vi "testRSASign&Verify.vi"(8 "error in (no error)":errorcluster, 11 "TestCase in":refnum<class "TestRSA.lvclass">) -> (0 "error out":errorcluster, 3 "TestCase out":refnum<class "TestRSA.lvclass">)   [LabVIEW 2021, in "TestRSA.lvclass"]
uses:
  TestRSA.lvclass
  TestRSA.lvclass/TestRSA.ctl
  <vilib>/addons/_JKI Toolkits/VI Tester/TestCase.llb/TestCase.lvclass
  Asymmetric Encryption/dotNET Crypto Asymmetric Encryption.lvlib
  Key Management/dotNET Crypto Key Management.lvlib
  Asymmetric Encryption/RSA/HashingAlgorithm.ctl
  Utility/dotNET Crypto Utility.lvlib
  Asymmetric Encryption/RSA/RSASignaturePadding.ctl
  C:/Program Files (x86)/National Instruments/LabVIEW 2021/vi.lib/addons/_JKI Toolkits/VI Tester/TestCase.llb/TestCase.lvclass
  C:/LabVIEW Working Directory/labview-keystore/Unit Tests/TestRSA/TestRSA.lvclass
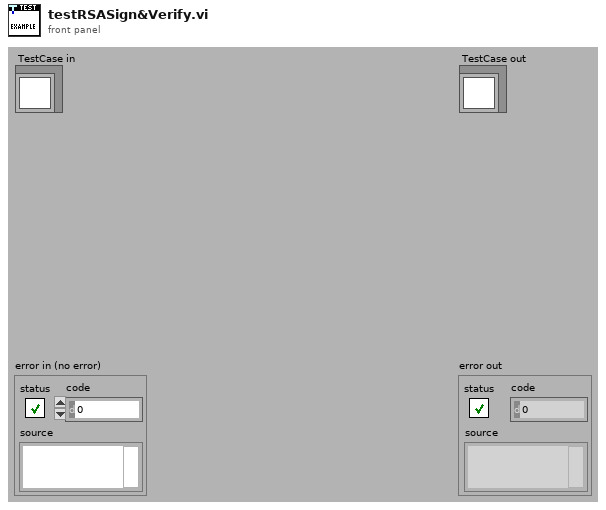
[diagram p1: front panel]
types:
  T1 = typedef "dotNET Crypto Asymmetric Encryption.lvlib/RSASignaturePadding.ctl" = enum16{"Pkcs1", "Pss"}
  T2 = typedef "dotNET Crypto Utility.lvlib/HashingAlgorithm.ctl" = enum16{"MD5", "SHA1", "SHA256", "SHA384", "SHA512"}
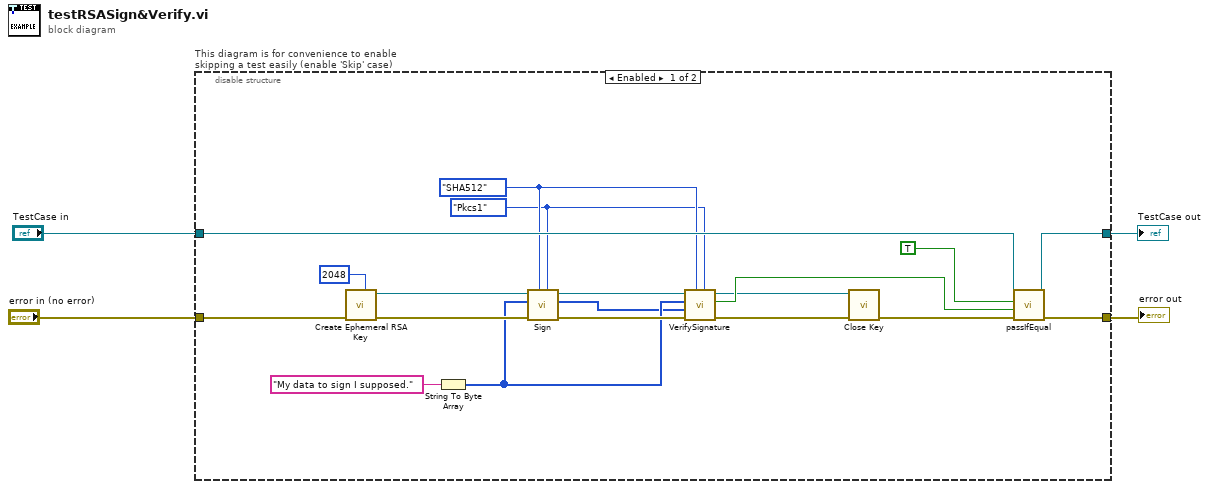
[diagram p0: block diagram]
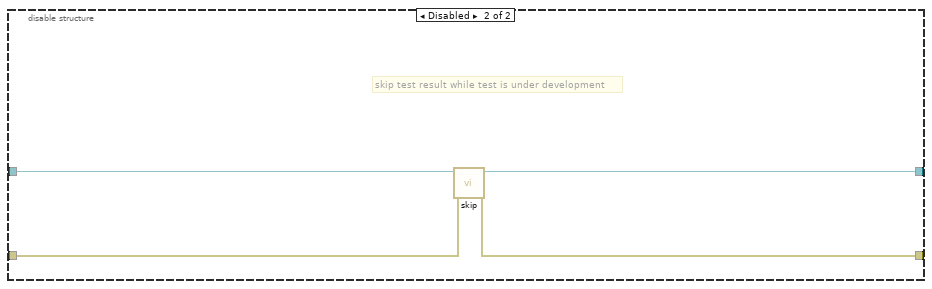
[diagram p2: hidden frame]
diagram:
  n1 = disable-structure "This diagram is for convenience to enable skipping a test easily (enable 'Skip' case)" shown="Enabled" {
    disable-tunnel: "TestCase in" -> [w23 w27]
    disable-tunnel: [w22 w25] -> w1
    disable-tunnel: [w21 w26] -> w3
    disable-tunnel: "error in (no error)" -> [w20 w24]
    frame Enabled {
      w16 = RSASignaturePadding."Pkcs1" ("RSASignPadding")
      w17 = HashingAlgorithm."SHA512" ("HashingAlgorithm")
      n2 = call "Create Ephemeral RSA Key.vi"("Key Length (2048)"=2048 ("keySize (2048 bit)"), "error in (no error)"=w20) -> ("error out"=w19:errorcluster, "CngKey out"=w12:refnum<k24>)  [unwired: 8 in]
      n3 = String To Byte Array(string="My data to sign I supposed.") -> (unsigned byte array=w11:u8[])
      n4 = call "Sign.vi"("RSASignPadding"=w16, "HashingAlgorithm"=w17, "error in (no error)"=w19, "Data in"=w11, "CngKey in"=w12) -> ("error out"=w18:errorcluster, "Signature out"=w10:u8[], "CngKey out"=w9:refnum<k24>)  [unwired: 4 in]
      n5 = call "VerifySignature.vi"("RSASignPadding"=w16, "HashingAlgorithm"=w17, "error in (no error)"=w18, "Signature in"=w10, "Data in"=w11, "CngKey in"=w9) -> ("error out"=w15:errorcluster, "Verified?"=w8:bool, "CngKey out"=w5:refnum<k24>)  [unwired: 3 in]
      n6 = call "Close Key.vi"("error in (no error)"=w15, "CngKey in"=w5) -> ("error out"=w6:errorcluster)  [unwired: 9 in]
      n7 = call-dynamic "passIfEqual.vi"("error in (no error)"=w6, "y"=w8, "x"=TRUE, "TestCase in"=w23) -> ("error out"=w21:errorcluster, "TestCase out"=w22:refnum<class "TestRSA.lvclass">)  [unwired: 6 in]
    }
    frame Disabled {
      # "skip test result while test is under development"
      n8 = call <vilib>:"skip.vi"("error in (no error)"=w24, "TestCase in"=w27) -> ("error out"=w26:errorcluster, "TestCase out"=w25:refnum<class "TestRSA.lvclass">)  [unwired: 8 in]
    }
  }
  "error out" <- w3
  "TestCase out" <- w1
